vi "Explanation Write.vi"(4 "error in (no error)":errorcluster, 5 "Value":string, 6 "Container State":T2, 7 "Display State In":T1) -> (0 "error out":errorcluster, 3 "Display State Out":T1)   [LabVIEW 2021, in "myRIO Choice Button.xctl"]
uses:
  <vilib>/myRIO/Common/Instrument Driver Framework/Utilities/xctls/myRIO Choice Button/myRIO Choice Button.xctl
  <vilib>/_xctls/Container State.ctl
  <vilib>/myRIO/Common/Instrument Driver Framework/Utilities/xctls/myRIO Choice Button/State.ctl
  <vilib>/_xctls/XControlSupport.lvlib
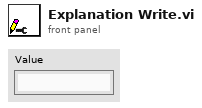
[diagram p1: front panel]
types:
  T1 = typedef "myRIO Choice Button.xctl/State.ctl" = cluster{"Title":string, "Explanation":string, "Mouse Enter Glyph":picture, "Mouse Down Glyph":picture, "Mouse Leave Glyph":picture, "Mouse Enter Background":picture, "Mouse Down Background":picture, "Mouse Leave Background":picture, "Button Mode":i32, "Button Square Frame":picture, "Disabled&GrayedOut":bool}
  T2 = typedef "XControlSupport.lvlib/Container State.ctl" = cluster{"Indicator?":bool, "Run Mode?":bool, " Refnum":refnum<vi>}
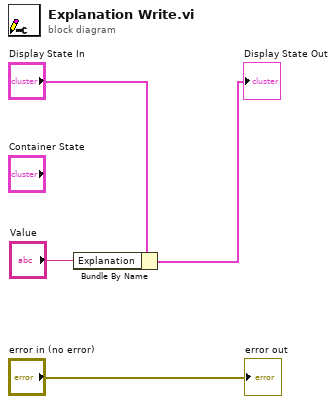
[diagram p0: block diagram]
diagram:
  n1 = Bundle By Name(cluster="Display State In", "Explanation"="Value") -> (→"Display State Out":T1)
  "error out" <- "error in (no error)"
